vi "Build CHM.vi"   [LabVIEW 2018]
uses:
  <vilib>/NI/Compiled HTML Menu Tool/CHM Generator/CHM Generator.lvclass
  <vilib>/Utility/config.llb/NI_LVConfig.lvlib
  <vilib>/Utility/config.llb/Read Key (String).vi
  <vilib>/Utility/config.llb/Read Key (Path).vi
types:
  T1 = typedef "NI_LVConfig.lvlib/Config Data RefNum.ctl" = refnum<k1>
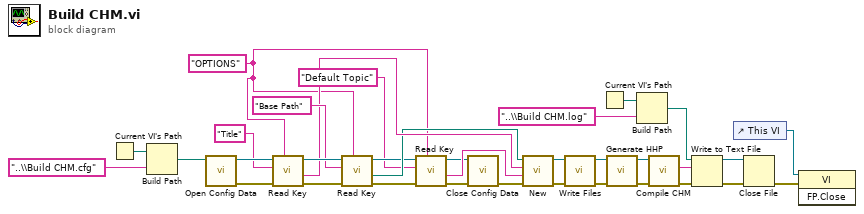
[diagram p0: block diagram]
diagram:
  w14 = "OPTIONS" ("section")
  n1 = Current VI's Path() -> (path=w13:path)
  n2 = Build Path(base path=w13, name or relative path="..\\Build CHM.cfg") -> (appended path=w11:path)
  n3 = call <vilib>:"Open Config Data.vi"("configuration file path"=w11) -> ("error out"=w27:errorcluster, "refnum"=w28:T1)  [unwired: 8 in, 1 out]
  n4 = call-poly <vilib>:"Read Key.vi"("section"=w14, "error in (no error)"=w27, "key"="Title", "refnum"=w28) -> ("error out"=w25:errorcluster, "value"=w22:string, "refnum out"=w24:T1)  [unwired: 4 in, 1 out]
  n5 = call-poly <vilib>:"Read Key.vi"("section"=w14, "error in (no error)"=w25, "key"="Base Path", "refnum"=w24) -> ("error out"=w21:errorcluster, "value"=w20:path, "refnum out"=w19:T1)  [unwired: 4 in, 1 out]
  n6 = call-poly <vilib>:"Read Key.vi"("section"=w14, "error in (no error)"=w21, "key"="Default Topic", "refnum"=w19) -> ("error out"=w16:errorcluster, "value"=w17:string, "refnum out"=w15:T1)  [unwired: 4 in, 1 out]
  n7 = call <vilib>:"Close Config Data.vi"("error in (no error)"=w16, "refnum"=w15) -> ("error out"=w2:errorcluster)  [unwired: 8 in, 1 out]
  n8 = call <vilib>:"New.vi"("error in (no error)"=w2, "Default topic"=w17, "Title"=w22, "Base Path"=w20) -> ("error out"=w33:errorcluster, "CHM Generator out"=w34:refnum<class "CHM Generator.lvclass">)  [unwired: 6 in]
  n9 = call-dynamic "Write Files.vi"("error in (no error)"=w33, "CHM Generator in"=w34) -> ("error out"=w32:errorcluster, "CHM Generator out"=w31:refnum<class "CHM Generator.lvclass">)  [unwired: 8 in]
  n10 = Current VI's Path() -> (path=w10:path)
  n11 = call-dynamic "Generate HHP.vi"("error in (no error)"=w32, "CHM Generator in"=w31) -> ("error out"=w29:errorcluster, "CHM Generator out"=w30:refnum<class "CHM Generator.lvclass">)  [unwired: 8 in]
  n12 = Build Path(base path=w10, name or relative path="..\\Build CHM.log") -> (appended path=w8:path)
  n13 = call <vilib>:"Compile CHM.vi"("error in (no error)"=w29, "CHM Generator in"=w30) -> ("error out"=w1:errorcluster, "standard output"=w7:string)  [unwired: 7 in, 1 out]
  n14 = Write to Text File(file (use dialog)=w8, text=w7, error in=w1) -> (refnum out=w5:refnum<file>, error out=w6:errorcluster)  [unwired: 1 in, 1 out]
  n15 = control-ref of="This VI"() -> (w4:refnum<vi>)
  n16 = Close File(refnum=w5, error in=w6) -> (error out=w3:errorcluster)  [unwired: 1 out]
  n17 = invoke class="VI" method="FP.Close"(reference=w4, error in=w3) -> ()  [unwired: 1 in, 3 out]
